vi "HGF_DSCSubscriber.AppendData2Variant.vi"(0 "variant":variant, 3 "Shared Variable":refnum<k21>, 4 "TypeDescriptor":string, 5 "error in":errorcluster) -> (14 "variant out":variant, 19 "error out":errorcluster)   [LabVIEW 2012, in "HGF_DSC.lvlib" / "HGF_DSCSubscriber.lvclass"]
uses:
  HGF_DSCSubscriber.lvclass
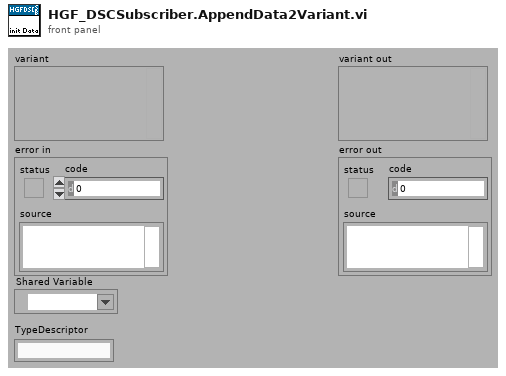
[diagram p1: front panel]
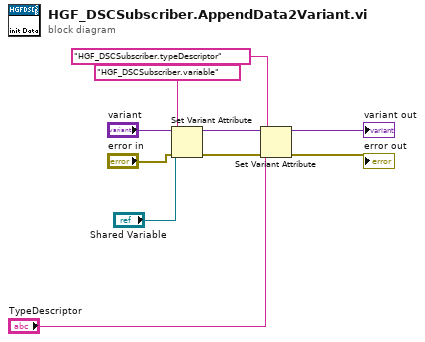
[diagram p0: block diagram]
diagram:
  n1 = Set Variant Attribute(Variant="variant", name="HGF_DSCSubscriber.variable", value="Shared Variable", error in="error in") -> (Variant out=w4:variant, error out=w6:errorcluster)  [unwired: 1 out]
  n2 = Set Variant Attribute(Variant=w4, name="HGF_DSCSubscriber.typeDescriptor", value="TypeDescriptor", error in=w6) -> (Variant out=→"variant out":variant, error out=→"error out":errorcluster)  [unwired: 1 out]
